vi "teste-circle.vi"() -> ()   [LabVIEW 2014]
panel:
  in  "Raio":dbl=0.5
  out "Y":dbl[](array[numeric])
  out "X":dbl[](array[numeric])
  in  "Y":dbl=2.0
  in  "X":dbl=2.0
  out "XY Graph":cluster{dbl[], dbl[]}(graph)
  in  "Density":dbl=100.0
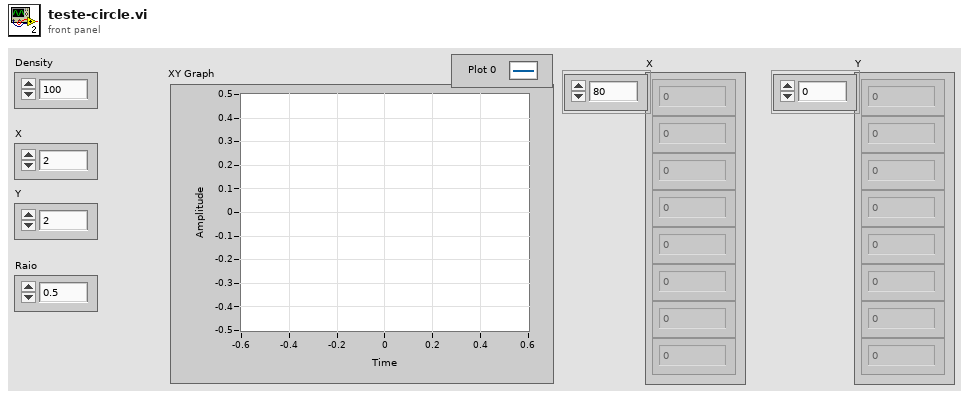
[diagram p1: front panel]
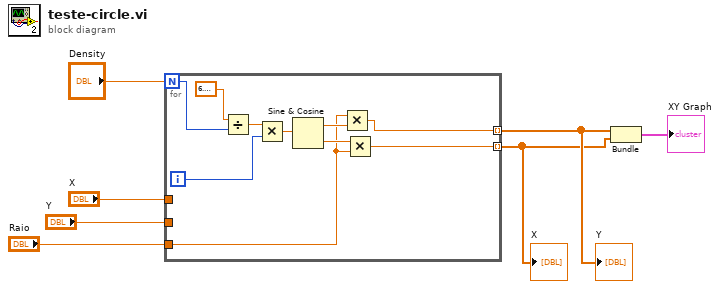
[diagram p0: block diagram]
diagram:
  n1 = for {
    N: "Density" -> [w12]
    tunnel: [w9] -> w7 mode=indexing
    tunnel: [w8] -> w6 mode=indexing
    tunnel: "X" -> [_]
    tunnel: "Y" -> [_]
    tunnel: "Raio" -> [w10]
    i -> [w11]
    n2 = Divide(x=6.283185307179586, y=w12) -> (x/y=w17:dbl)
    n3 = Multiply(x=w17, y=w11) -> (x*y=w16:dbl)
    n4 = Sine & Cosine(0:w16) -> (1:w15:dbl, 2:w14:dbl)
    n5 = Multiply(x=w10, y=w15) -> (x*y=w9:dbl)
    n6 = Multiply(x=w14, y=w10) -> (x*y=w8:dbl)
  }
  "X" <- w6
  "Y" <- w7
  n7 = Bundle(w7, w6) -> (→"XY Graph":cluster{dbl[], dbl[]})  [unwired: 1 in]
